vi "Eucledian Distance.vi"(8 "Y2":dbl, 9 "X2":dbl, 10 "Y":dbl, 11 "X":dbl) -> (2 "Distance":dbl)   [LabVIEW 2017]
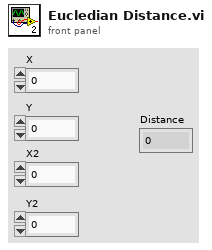
[diagram p1: front panel]
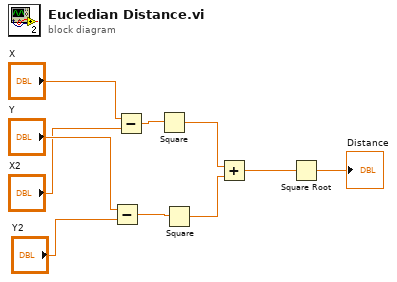
[diagram p0: block diagram]
diagram:
  n1 = Subtract(x="Y", y="Y2") -> (x-y=w5:dbl)
  n2 = Subtract(x="X", y="X2") -> (x-y=w6:dbl)
  n3 = Square(x=w6) -> (x^2=w4:dbl)
  n4 = Square(x=w5) -> (x^2=w3:dbl)
  n5 = Add(x=w4, y=w3) -> (x+y=w1:dbl)
  n6 = Square Root(x=w1) -> (sqrt(x)=→"Distance":dbl)
